vi "CMN_GetSpecificArg.vi"(8 "error in (no error)":errorcluster, 9 "key name":string, 10 "command list":string) -> (0 "error out":errorcluster, 2 "value":string)   [LabVIEW 2016]
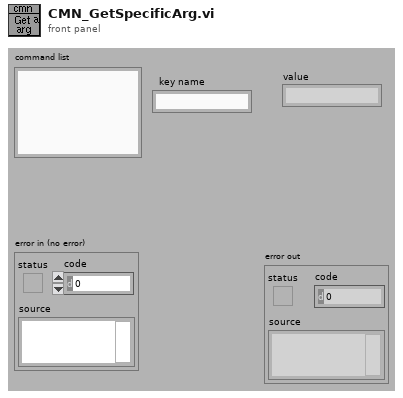
[diagram p1: front panel]
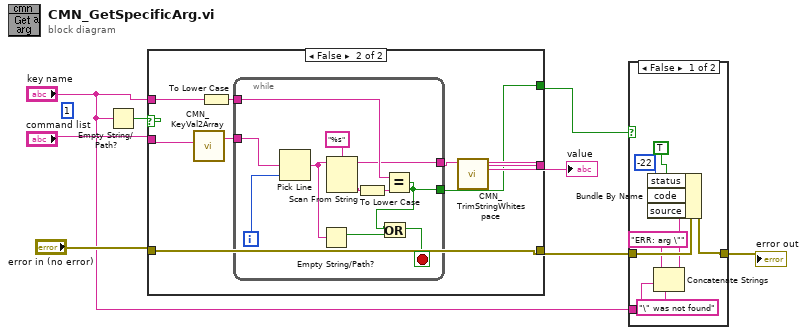
[diagram p0: block diagram]
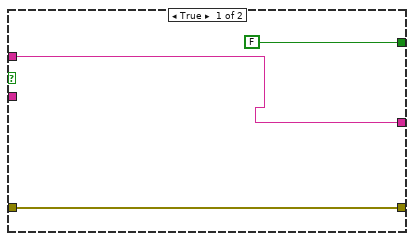
[diagram p3: hidden frame]
diagram:
  (unwired) 1
  n1 = Empty String/Path?(string/path="key name") -> (empty?=w6:bool)
  n2 = case shown="False" w6 {
    tunnel: "command list" -> [_ w12]
    tunnel: "key name" -> [w11 w19]
    tunnel: [w11 w16] -> w7
    tunnel: "error in (no error)" -> [w9 w15]
    tunnel: [w9 w15] -> w4
    tunnel: [FALSE w14] -> w2
    frame True {
    }
    frame False {
      n3 = call "CMN_KeyVal2Array.vi"("command in"=w12) -> ("commands out"=w13:string)  [unwired: 2 in, 7 out]
      n4 = To Lower Case(string=w19) -> (all lower case string=w18:string)
      n5 = while {
        tunnel: w13 -> [w21]
        tunnel: w18 -> [w26]
        tunnel: [w24] -> w14
        tunnel: [w23] -> w17
        i -> [w22]
        stop <- w30 stop-if-true
        n6 = Pick Line(multi-line string=w21, line index=w22) -> (output string=w29:string)  [unwired: 1 out]
        n7 = Empty String/Path?(string/path=w29) -> (empty?=w25:bool)
        n8 = Scan From String(format string="%s", input string=w29) -> (remaining string=w23:string, output 1=w27:string)  [unwired: 2 in, 3 out]
        n9 = To Lower Case(string=w27) -> (all lower case string=w20:string)
        n10 = Equal?(x=w26, y=w20) -> (x = y?=w24:bool)
        n11 = Or(x=w24, y=w25) -> (x .or. y?=w30:bool)
      }
      n12 = call "CMN_TrimStringWhitespace.vi"("string"=w17) -> ("trimmed string"=w16:string)  [unwired: 1 in, 8 out]
    }
  }
  "value" <- w7
  n13 = case shown="False" w2 {
    tunnel: w4 -> [w37 w39]
    tunnel: [w36 w39] -> w3
    tunnel: "key name" -> [w33 _]
    frame False {
      n14 = Concatenate Strings("ERR: arg \"" ("source"), w33, "\" was not found" ("string")) -> (w31:string)
      n15 = Bundle By Name(cluster=w37, "status"=TRUE, "code"=-22, "source"=w31) -> (w36:errorcluster)
    }
    frame True {
    }
  }
  "error out" <- w3
